vi "OE 1c Sum using While.vi"() -> ()   [LabVIEW 2021]
panel:
  in  "?":string
  in  "?":string
  in  "Input":dbl
  out "Numeric":i32
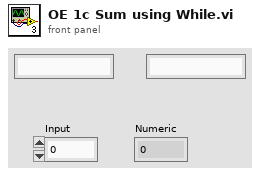
[diagram p1: front panel]
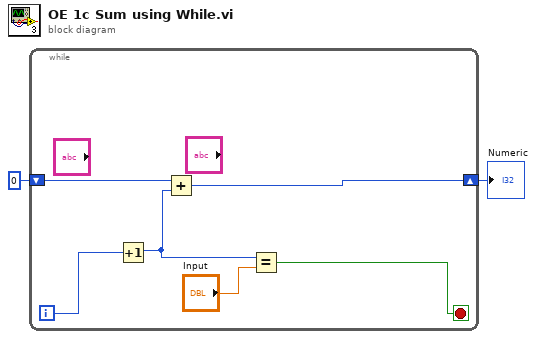
[diagram p0: block diagram]
diagram:
  n1 = while {
    shift-right: [w6] -> w1
    shift-left: 0 -> [w7]
    i -> [w8]
    stop <- w3 stop-if-true
    n2 = Increment(x=w8) -> (x+1=w4:i32)
    n3 = Add(x=w7, y=w4) -> (x+y=w6:i32)
    n4 = Equal?(x=w4, y="Input") -> (x = y?=w3:bool)
  }
  "Numeric" <- w1
